vi "Read Buffer.vi"(6 "data length (32)":u8=32, 8 "error in":errorcluster, 9 "buffer type":T1(ring)=enum."BC Message Buffer", 10 "buffer id":u16=1, 11 "module handle":u32) -> (0 "error out":errorcluster, 1 "data buffer index":u16, 2 "data array out":u16[](array[numeric]), 3 "module handle out":u32)   [LabVIEW 2020, in "AIM MIL-STD-1553 Hardware API.lvlib"]
uses:
  AIM MIL-STD-1553 Hardware API.lvlib
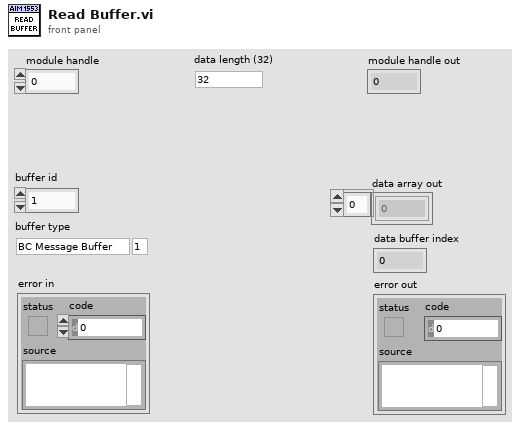
[diagram p1: front panel]
types:
  T1 = enum16{"unknown", "BC Message Buffer", "RT Message Buffer"}
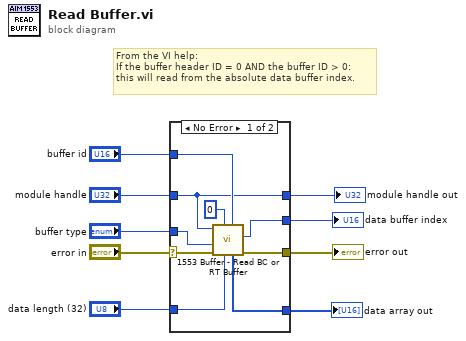
[diagram p0: block diagram]
diagram:
  # "From the VI help:\nIf the buffer header ID = 0 AND the buffer ID > 0:\nthis will read from the absolute data buffer index."
  n1 = case shown="No Error" "error in" {
    selector: "error in" -> [w18 w20]
    tunnel: [w15 w20] -> w9
    tunnel: "module handle" -> [w10 w19]
    tunnel: "buffer type" -> [w17 _]
    tunnel: "buffer id" -> [w12 _]
    tunnel: "data length (32)" -> [w16 _]
    tunnel: [w14 _] -> w4
    tunnel: [w13 _] -> w3
    tunnel: [w10 w19] -> w1
    frame No Error {
      n2 = call <instrlib>:"1553 Buffer - Read BC or RT Buffer.vi"("Buffer ID (1)"=w12, "Data Length (32)"=w16, "Buffer Header ID (1)"=u16 0, "Error In (none)"=w18, "Buffer Type (BC)"=w17, "Module Handle"=w10) -> ("Error Out"=w15:errorcluster, "Data Buffer Index"=w13:u16, "Data Array Out"=w14:u16[])  [unwired: 2 in, 1 out]
    }
    frame Error {
    }
  }
  "error out" <- w9
  "data array out" <- w4
  "data buffer index" <- w3
  "module handle out" <- w1
